vi "Example_BP Network_Classification.vi"() -> ()   [LabVIEW 2009]
uses:
  <vilib>/addons/Machine Learning/Supervised Learning/ml_BP_Terminal Condition.ctl
  <vilib>/Utility/miscctls.llb/LV3DPointTypeDef.ctl
  <vilib>/addons/Machine Learning/Visualization/Visualization (3D).vi
  <vilib>/addons/Machine Learning/Utilities/Training & Test Set (matrix-class).vi
  <vilib>/addons/Machine Learning/NILabs_MLT.lvlib
panel:
  in  "Data set":enum16{"4 Gaussians", "3 Concentric Circles"}(ring)
  out "Classification accuracy":dbl
  out "Test data":refnum<vi>(3d-picture)
  in  "Stopping criteria":T1={"min MSE"=1e-05, "min delta MSE"=1e-08, "min step length"=1e-08, "max iteration"=1000.0}
  in  "# of hidden neurons":i32=5
  out "Training data":refnum<vi>(3d-picture)
  out "Training MSE":dbl
  # "Introduction:\nA Back-propagation (BP) neural network is applied to two classification problems."
  # "%"
  # "(Samples are overlain with class labels predicted by the BP network.)"
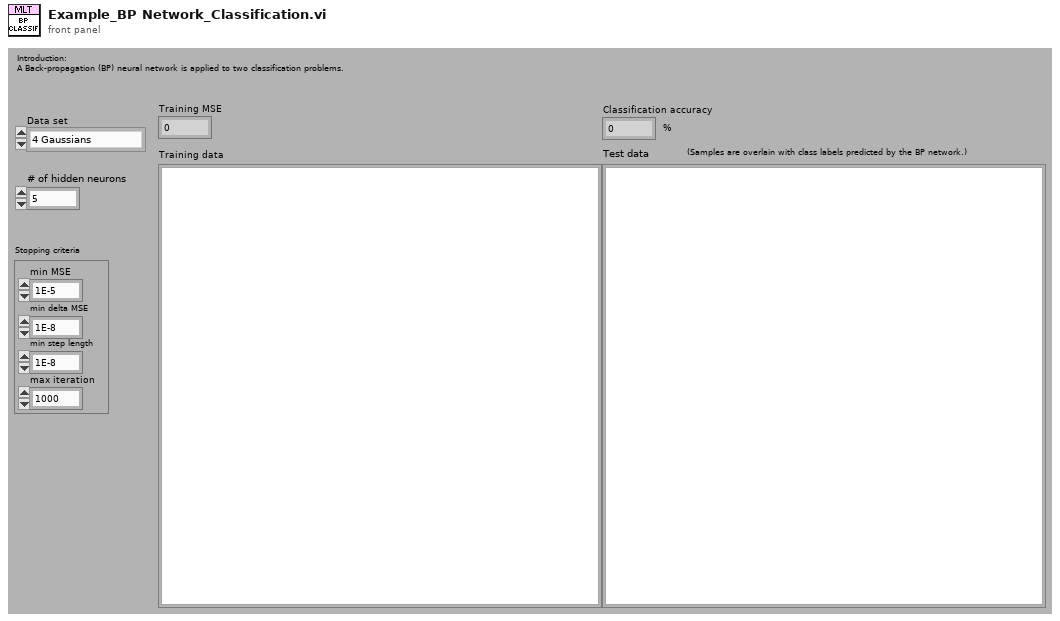
[diagram p1: front panel]
types:
  T1 = typedef "NILabs_MLT.lvlib/ml_BP_Terminal Condition.ctl" = cluster{"min MSE":dbl, "min delta MSE":dbl, "min step length":dbl, "max iteration":dbl}
  T2 = typedef "LV3DPointTypeDef.ctl" = cluster{"X":sgl, "Y":sgl, "Z":sgl}
  T3 = typedef "NILabs_MLT.lvlib/ml_BP_Project.ctl" = cluster{"Training Data":T4, "Normalize Info":T5, "3-layer NN":T6, "Ternimal Condition":T1}
  T4 = typedef "NILabs_MLT.lvlib/ml_BP_Data.ctl" = cluster{"dim in":i32, "dim out":i32, "# samples":i32, "Input":dbl[][], "Output":dbl[][]}
  T5 = typedef "NILabs_MLT.lvlib/ml_BP_Normalize Data.ctl" = cluster{"input min":dbl[], "input max":dbl[], "output min":dbl[], "output max":dbl[]}
  T6 = typedef "NILabs_MLT.lvlib/ml_BP_3layer Feedforward.ctl" = cluster{"# input neuron ":i32, "# hidden neuron":i32, "# output neuron":i32, "Weight (I->H)":dbl[][], "Weight (H->O)":dbl[][], "Output":dbl[][], "Hidden Out":dbl[][], "Derivation Output":dbl[][], "Derivation Hidden":dbl[][], "dw (I->H)":dbl[][], "dw (H->O)":dbl[][]}
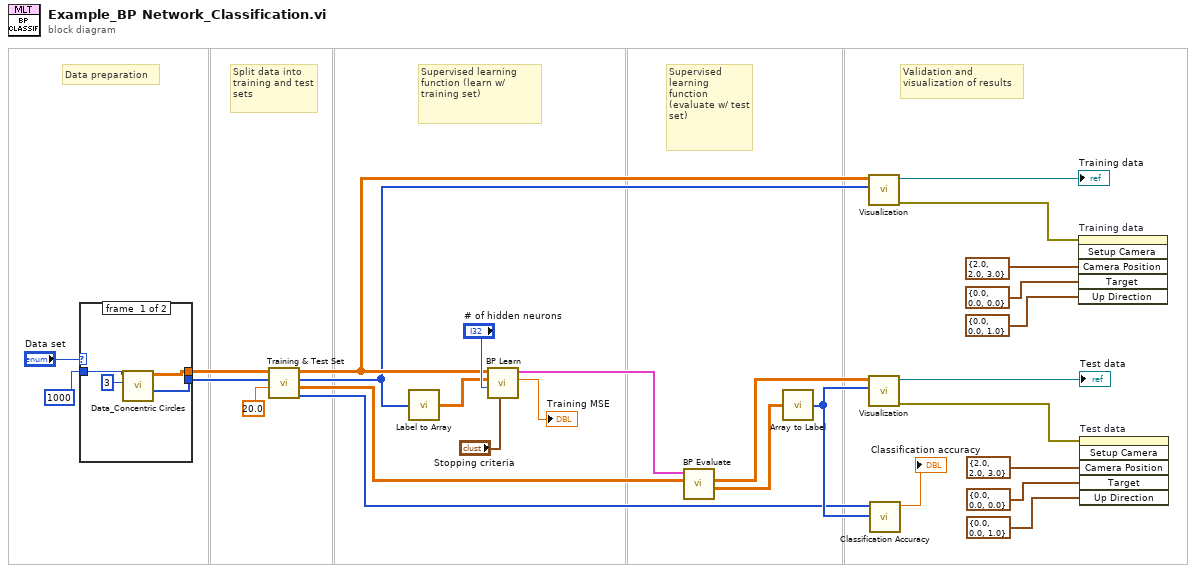
[diagram p0: block diagram]
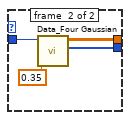
[diagram p2: hidden frame]
diagram:
  # "Validation and visualization of results"
  # "Supervised learning function (evaluate w/ test set)"
  # "Supervised learning function (learn w/ training set)"
  # "Split data into training and test sets"
  # "Data preparation"
  n1 = case shown="\"3 Concentric Circles\"" "Data set" {
    tunnel: [w30 w36] -> w28
    tunnel: 1000 ("# of points") -> [w32 w35]
    tunnel: [w29 w34] -> w17
    frame #0 {
      n2 = call "Data_Concentric Circles.vi"("# of circles"=3, "# of points"=w32) -> ("Classes"=w29:i32[], "Data"=w30:dbl[][])  [unwired: 8 in]
    }
    frame #1 {
      n3 = call "Data_Four Gaussian.vi"("noise amplitude"=0.35, "# of points"=w35) -> ("Classes"=w34:i32[], "Data"=w36:dbl[][])  [unwired: 8 in]
    }
  }
  n4 = call-poly <vilib>:"Training & Test Set.vi"("percent"=20.0, "classes"=w17, "Samples"=w28) -> ("Test Set classes"=w3:i32[], "Test Set Data"=w23:dbl[][], "Training Set classes"=w14:i32[], "Training Set Data"=w15:dbl[][])  [unwired: 5 in]
  n5 = call <vilib>:"Label to Array.vi"("Classes"=w14) -> ("Array"=w16:dbl[][])  [unwired: 1 in]
  n6 = call <vilib>:"BP Learn.vi"("Stopping Criteria"="Stopping criteria", "# of hidden neuron"="# of hidden neurons", "Training outputs"=w16, "Training data samples"=w15) -> ("mse"=→"Training MSE":dbl, "BP Project"=w24:T3)  [unwired: 4 in, 2 out]
  n7 = call <vilib>:"BP Evaluate.vi"("Test data samples"=w23, "BP Project"=w24) -> ("NN outputs"=w7:dbl[][], "Test data samples dup"=w8:dbl[][])  [unwired: 5 in, 3 out]
  n8 = call <vilib>:"Array to Label.vi"("Array"=w7) -> ("Classes"=w4:i32[])
  n9 = call-poly <vilib>:"Visualization.vi"("Class labels"=w14, "Data samples"=w15) -> ("error out"=w18:errorcluster, "3D Picture"=→"Training data":refnum<vi>)  [unwired: 8 in]
  n10 = call-poly <vilib>:"Visualization.vi"("Class labels"=w4, "Data samples"=w8) -> ("error out"=w13:errorcluster, "3D Picture"=→"Test data":refnum<vi>)  [unwired: 8 in]
  n11 = call <vilib>:"Classification Accuracy.vi"("Predicted class labels"=w4, "Actual class labels"=w3) -> ("Classification Accuracy"=→"Classification accuracy":dbl)  [unwired: 8 in, 1 out]
  n12 = invoke on="Training data" class="SceneGraphDisp (strict)" method="Setup Camera"(error in=w18, "Camera Position"=T2 {"X"=2.0, "Y"=2.0, "Z"=3.0}, "Target"=T2 {"X"=0.0, "Y"=0.0, "Z"=0.0} ("Camera Position"), "Up Direction"=T2 {"X"=0.0, "Y"=0.0, "Z"=1.0} ("Camera Position")) -> ()  [unwired: 2 in, 6 out]
  n13 = invoke on="Test data" class="SceneGraphDisp (strict)" method="Setup Camera"(error in=w13, "Camera Position"=T2 {"X"=2.0, "Y"=2.0, "Z"=3.0}, "Target"=T2 {"X"=0.0, "Y"=0.0, "Z"=0.0} ("Camera Position"), "Up Direction"=T2 {"X"=0.0, "Y"=0.0, "Z"=1.0} ("Camera Position")) -> ()  [unwired: 2 in, 6 out]
